vi "Voltage_Multiple_Measurements.vi"() -> ()   [LabVIEW 2013]
uses:
  <vilib>/Analysis/baseanly.llb/Mean (DBL).vi
  <vilib>/Utility/file.llb/Write To Spreadsheet File (DBL).vi
  <vilib>/Analysis/NI_AALBase.lvlib
panel:
  in  "Write report":bool
  in  "File path":path
  out "Voltage Array":dbl[](array[numeric])
  out "Average Value, V":dbl
  out "Min Value, V":dbl
  out "Max Value, V":dbl
  in  "Number of samples":i32
  out "Voltage Graph":dbl[](graph)
  out "Voltage Chart":dbl(graph)
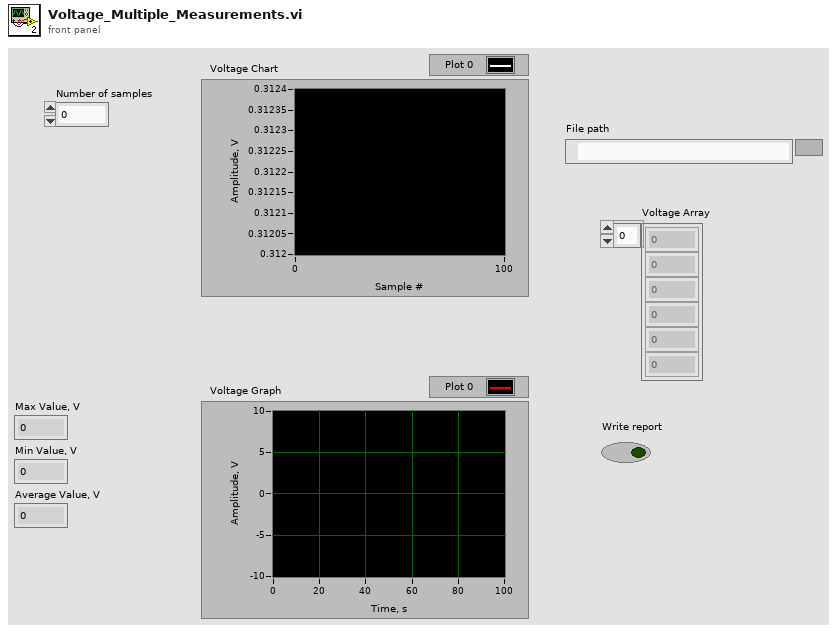
[diagram p1: front panel]
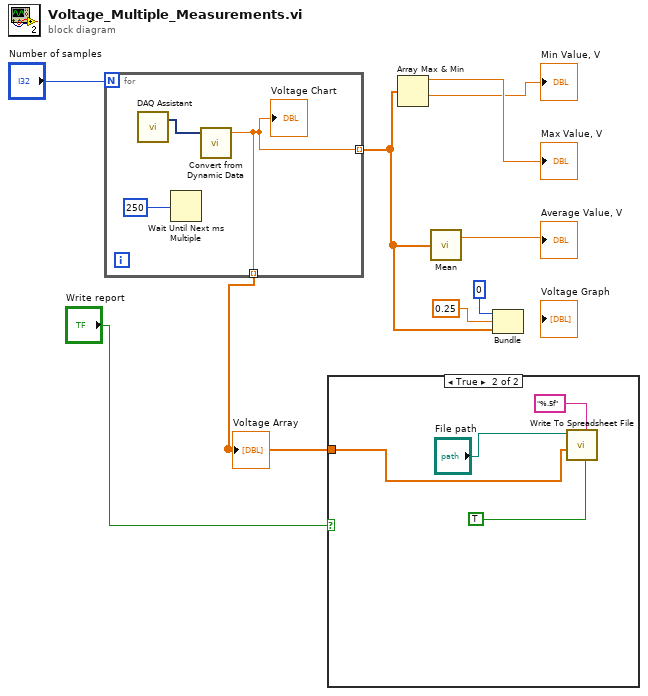
[diagram p0: block diagram]
diagram:
  n1 = for {
    N: "Number of samples" -> [_]
    tunnel: [w10] -> w5 mode=indexing
    tunnel: [w10] -> w1 mode=indexing
    n2 = call "DAQ Assistant"() -> ("data"=w11:dynamicdata)  [unwired: 17 in, 2 out]
    n3 = Wait Until Next ms Multiple(millisecond multiple=250) -> ()  [unwired: 1 out]
    n4 = call "Convert from Dynamic Data"("Dynamic Data Type"=w11) -> ("Scalar"=w10:dbl)  [unwired: 3 in]
    "Voltage Chart" <- w10
  }
  "Voltage Array" <- w1
  n5 = case shown="True" "Write report" {
    tunnel: w1 -> [_ w15]
    frame False {
    }
    frame True {
      n6 = call-poly <vilib>:"Write To Spreadsheet File.vi"("transpose? (no:F)"=TRUE, "format (%.3f)"="%.5f", "1D data"=w15, "file path (dialog if empty)"="File path") -> ()  [unwired: 4 in, 1 out]
    }
  }
  n7 = Array Max & Min(array=w5) -> (max value=→"Max Value, V":dbl, min value=→"Min Value, V":dbl)  [unwired: 2 out]
  n8 = call-poly <vilib>:"Mean.vi"("X"=w5) -> ("mean"=→"Average Value, V":dbl)  [unwired: 1 out]
  n9 = Bundle(0, 0.25, w5) -> ()  [unwired: 1 in, 1 out]
